vi "Template change for pattern match.vi"() -> ()   [LabVIEW 2011]
panel:
  out "Template for Encapsulation pattern matching":path
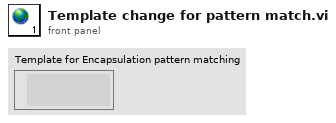
[diagram p1: front panel]
diagram:
